vi "IOR4 Relay Control .vi"(7 "Relay Control Sequence":T1(array[ring]), 8 "error in (no error)":errorcluster, 10 "#Writes per cmd":enum16{"1", "2", "3", "4", "5"}(ring)=enum."2", 11 "Relay ComPort":refnum<visa-resource-name>) -> (0 "error out":errorcluster)   [LabVIEW 2020, in "DLP Design Modules Driver.lvlib"]
uses:
  <vilib>/Instr/_visa.llb/VISA Configure Serial Port (Instr).vi
  DLP Design Modules Driver.lvlib
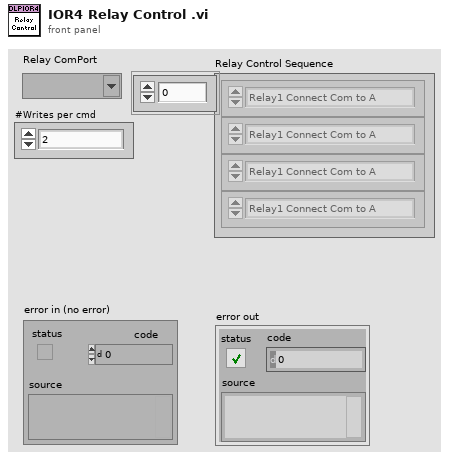
[diagram p1: front panel]
types:
  T1 = enum16{"Relay1 Connect Com to A", "Relay1 Connect Com to B", "Relay2 Connect Com to A", "Relay2 Connect Com to B", "Relay3 Connect Com to A", "Relay3 Connect Com to B", "Relay4 Connect Com to A", "Relay4 Connect Com to B"}[]
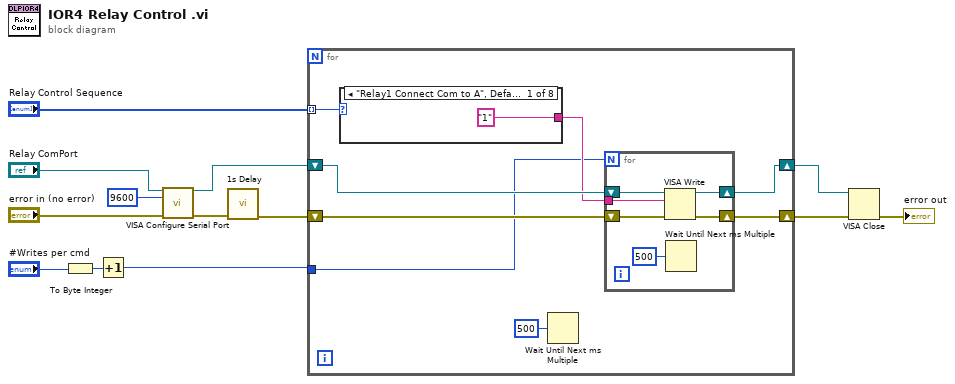
[diagram p0: block diagram]
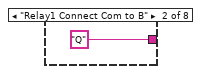
[diagram p2: hidden frame]
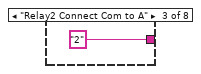
[diagram p3: hidden frame]
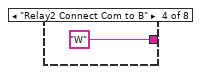
[diagram p4: hidden frame]
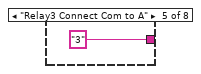
[diagram p5: hidden frame]
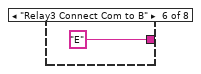
[diagram p6: hidden frame]
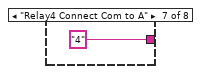
[diagram p7: hidden frame]
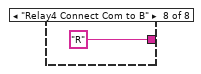
[diagram p8: hidden frame]
diagram:
  n1 = To Byte Integer(number="#Writes per cmd") -> (8bit integer=w1:i8)
  n2 = Increment(x=w1) -> (x+1=w3:i8)
  n3 = call-poly "VISA Configure Serial Port"("VISA resource name"="Relay ComPort", "baud rate (9600)"=u32 9600, "error in (no error)"="error in (no error)") -> ("VISA resource name out"=w8:refnum<visa-resource-name>, "error out"=w10:errorcluster)  [unwired: 11 in]
  n4 = call "1s Delay"("error in (no error)"=w10) -> ("error out"=w9:errorcluster)  [unwired: 10 in]
  n5 = for {
    tunnel: "Relay Control Sequence" -> [w19] mode=indexing
    shift-right: [w17] -> w5
    shift-left: w8 -> [w20]
    shift-right: [w16] -> w6
    shift-left: w9 -> [w21]
    tunnel: w3 -> [w15]
    n6 = case shown="\"Relay1 Connect Com to A\", Default" w19 {
      tunnel: ["1" ("write buffer") "Q" ("write buffer") "2" ("write buffer") "W" ("write buffer") "3" ("write buffer") "E" ("write buffer") "4" ("write buffer") "R" ("write buffer")] -> w18
      frame "Relay1 Connect Com to A", Default {
      }
      frame "Relay1 Connect Com to B" {
      }
      frame "Relay2 Connect Com to A" {
      }
      frame "Relay2 Connect Com to B" {
      }
      frame "Relay3 Connect Com to A" {
      }
      frame "Relay3 Connect Com to B" {
      }
      frame "Relay4 Connect Com to A" {
      }
      frame "Relay4 Connect Com to B" {
      }
    }
    n7 = Wait Until Next ms Multiple(millisecond multiple=u32 500) -> ()  [unwired: 1 out]
    n8 = for {
      N: w15 -> [_]
      tunnel: w18 -> [w24]
      shift-right: [w22] -> w16
      shift-left: w21 -> [w27]
      shift-right: [w23] -> w17
      shift-left: w20 -> [w26]
      n9 = VISA Write(VISA resource name=w26, write buffer=w24, error in (no error)=w27) -> (VISA resource name out=w23:refnum<visa-resource-name>, error out=w22:errorcluster)  [unwired: 1 out]
      n10 = Wait Until Next ms Multiple(millisecond multiple=u32 500) -> ()  [unwired: 1 out]
    }
  }
  n11 = VISA Close(VISA resource name=w5, error in (no error)=w6) -> (error out=→"error out":errorcluster)
